vi "Read N attempt.vi"(8 "error in (no error)":errorcluster, 11 "MB_TCP in":refnum<class "MB_TCP.lvclass">) -> (0 "error out":errorcluster, 2 "N attempt":i32, 3 "MB_TCP out":refnum<class "MB_TCP.lvclass">)   [LabVIEW 2021, in "MB_TCP.lvclass"]
uses:
  MB_TCP.lvclass
  MB_TCP.lvclass/MB_TCP.ctl
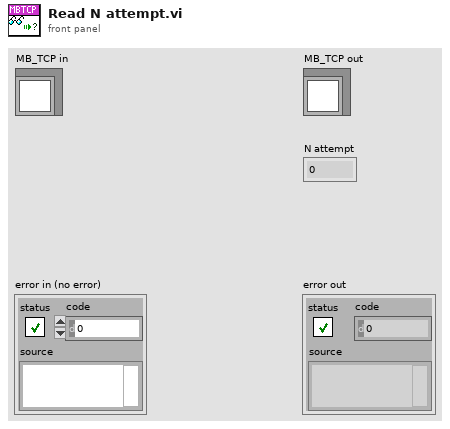
[diagram p1: front panel]
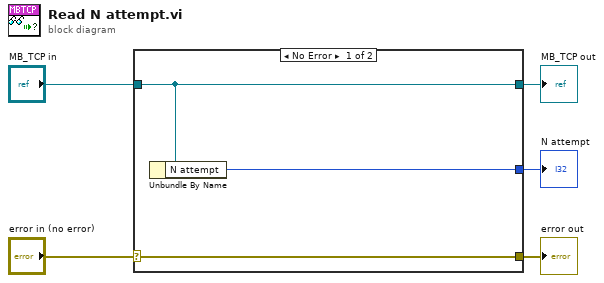
[diagram p0: block diagram]
diagram:
  n1 = case shown="No Error" "error in (no error)" {
    selector: "error in (no error)" -> [w8 w9]
    tunnel: [w8 w9] -> w4
    tunnel: [w7 w10] -> w2
    tunnel: "MB_TCP in" -> [w7 w10]
    tunnel: [w6 _] -> w1
    frame No Error {
      n2 = Unbundle By Name(w7) -> ("N attempt"=w6:i32)
    }
    frame Error {
    }
  }
  "error out" <- w4
  "MB_TCP out" <- w2
  "N attempt" <- w1
